vi "GetUint8Be.vi"(4 "错误输入":errorcluster, 7 "refnum in":refnum<file>) -> (0 "错误输出":errorcluster, 2 "uint8":u8, 3 "refnum out":refnum<file>)   [LabVIEW 2016]
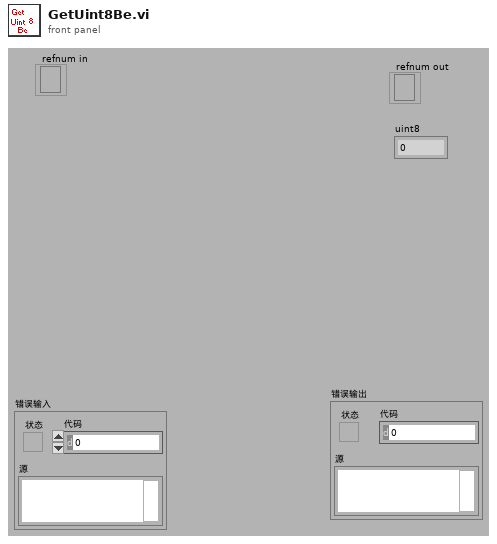
[diagram p1: front panel]
types:
  T1 = enum16{"big-endian, network order", "native, host order", "little-endian"}
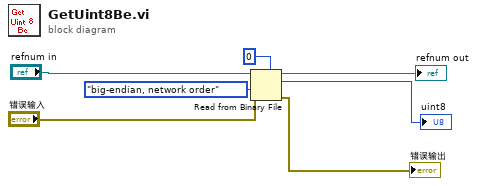
[diagram p0: block diagram]
diagram:
  n1 = Read from Binary File(5:u8 0 ("总数(1)"), 8:"错误输入", 9:T1."big-endian, network order" ("字节顺序(0:big-endian, network order)"), 11:"refnum in") -> (0:→"错误输出":errorcluster, 2:→"uint8":u8, 3:→"refnum out":refnum<file>)  [unwired: 3 out]
